vi "ADXL_convert_to_g.vi"(2 "volts-to-g conversion factor (0.3V/g) for ADXL335":dbl=0.3 format="%#_13g", 3 "center value (0g)":dbl=1.7 format="%#_13g", 4 "system power (Volts)":dbl=3.3 format="%#_13g", 5 "ADXL analog data out: Binary format":u16[][](array[numeric])) -> (0 "accelvolts":dbl[][](array[numeric]), 1 "ADXL scaled (units of g)":dbl[][](array[numeric]))   [LabVIEW 2020]
panel:
  out "calibration factor":ext
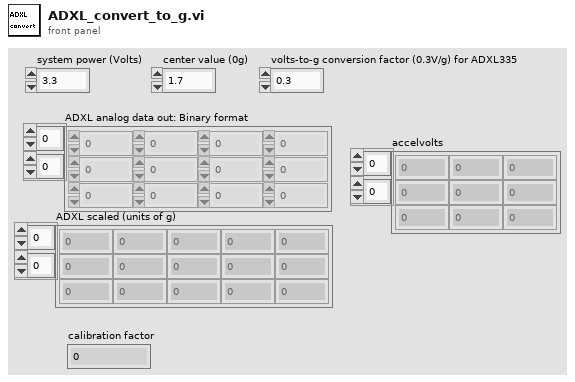
[diagram p1: front panel]
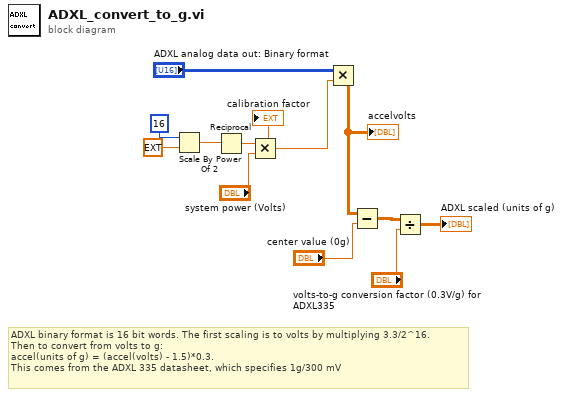
[diagram p0: block diagram]
diagram:
  # "ADXL binary format is 16 bit words. The first scaling is to volts by multiplying 3.3/2^16.\nThen to convert from volts to g:\naccel(units of g) = (accel(volts) - 1.5)*0.3.\nThis comes from the ADXL 335 datasheet, which specifies 1g/300 mV"
  n1 = Scale By Power Of 2(n=i16 16, x=ext 1.0) -> (x*2^n=w8:ext)
  n2 = Reciprocal(x=w8) -> (1/x=w7:ext)
  n3 = Multiply(x=w7, y="system power (Volts)") -> (x*y=w5:ext)
  "calibration factor" <- w5
  n4 = Multiply(x="ADXL analog data out: Binary format", y=w5) -> (x*y=w4:ext[][])
  "accelvolts" <- w4
  n5 = Subtract(x=w4, y="center value (0g)") -> (x-y=w11:ext[][])
  n6 = Divide(x=w11, y="volts-to-g conversion factor (0.3V/g) for ADXL335") -> (x/y=→"ADXL scaled (units of g)":ext[][])
